vi "initCAN2.vi"(2 "BaudRate":u32=1000000, 3 "SlotNum":u32, 4 "CAN":cluster{"Interface":refnum<k21>[], "Slot":u32[]}) -> (0 "session write":refnum<k21>, 1 "session read":refnum<k21>)   [LabVIEW 2018]
uses:
  <vilib>/xnet/xnet.llb/XNET Create Session (Frame Input Stream).vi
  <vilib>/xnet/xnet.llb/XNET Create Session (Frame Output Stream).vi
  <resource>/objmgr/xnet.rc
panel:
  out "error out":errorcluster
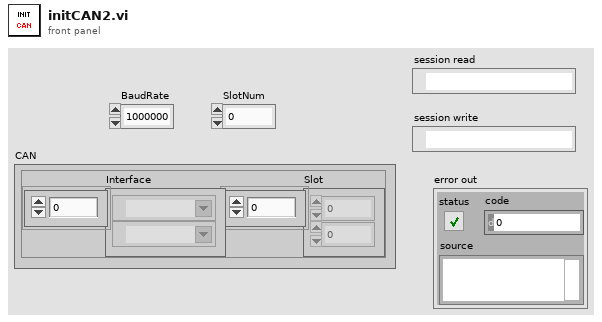
[diagram p1: front panel]
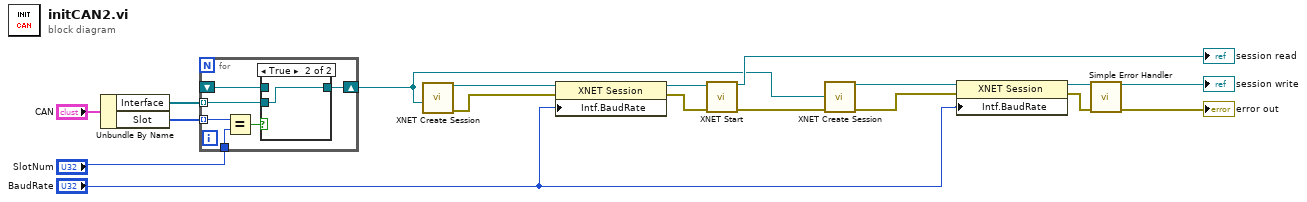
[diagram p0: block diagram]
diagram:
  n1 = Unbundle By Name("CAN") -> ("Interface"=w4:refnum<k21>[], "Slot"=w5:u32[])
  n2 = for {
    tunnel: w5 -> [w23] mode=indexing
    tunnel: w4 -> [w21] mode=indexing
    shift-right: [w20] -> w2
    shift-left: _ -> [w19]
    tunnel: "SlotNum" -> [w18]
    n3 = Equal?(x=w23, y=w18) -> (x = y?=w22:bool)
    n4 = case shown="True" w22 {
      tunnel: w21 -> [_ w25]
      tunnel: [w24 w25] -> w20
      tunnel: w19 -> [w24 _]
      frame False {
      }
      frame True {
      }
    }
  }
  n5 = call-poly <vilib>:"XNET Create Session.vi"("interface"=w2) -> ("session out"=w15:refnum<k21>, "error out"=w16:errorcluster)  [unwired: 2 in, 11 out]
  n6 = property class="XNET Session"(reference=w15, error in=w16, "Intf.BaudRate"="BaudRate") -> (reference out=w13:refnum<k21>, error out=w12:errorcluster)
  n7 = call <vilib>:"XNET Start.vi"("session in"=w13, "error in (no error)"=w12) -> ("session out"=→"session read":refnum<k21>, "error out"=w11:errorcluster)  [unwired: 12 out]
  n8 = call-poly <vilib>:"XNET Create Session.vi"("interface"=w2, "error in (no error)"=w11) -> ("session out"=w17:refnum<k21>, "error out"=w10:errorcluster)  [unwired: 1 in, 11 out]
  n9 = property class="XNET Session"(reference=w17, error in=w10, "Intf.BaudRate"="BaudRate") -> (reference out=→"session write":refnum<k21>, error out=w14:errorcluster)
  n10 = call <vilib>:"Simple Error Handler.vi"("error in (no error)"=w14) -> ("error out"=→"error out":errorcluster)  [unwired: 4 in, 4 out]
